vi "Modify_Dot_Characterstic(Status)-2.vi"(0 "Dot matrix IN":i16[][](array[numeric]), 1 "X2":dbl, 2 "Y2":dbl, 5 "Frame-to-frame displ":dbl[][](array[numeric]), 7 "Dot charact":i16, 9 "multipler":i32=4, 11 "error IN":errorcluster, 12 "# column":i32, 13 "Size Rows":i32) -> (4 "Dot matrix OUT":i16[][](array[numeric]), 15 "error OUT":errorcluster)   [LabVIEW 2013]
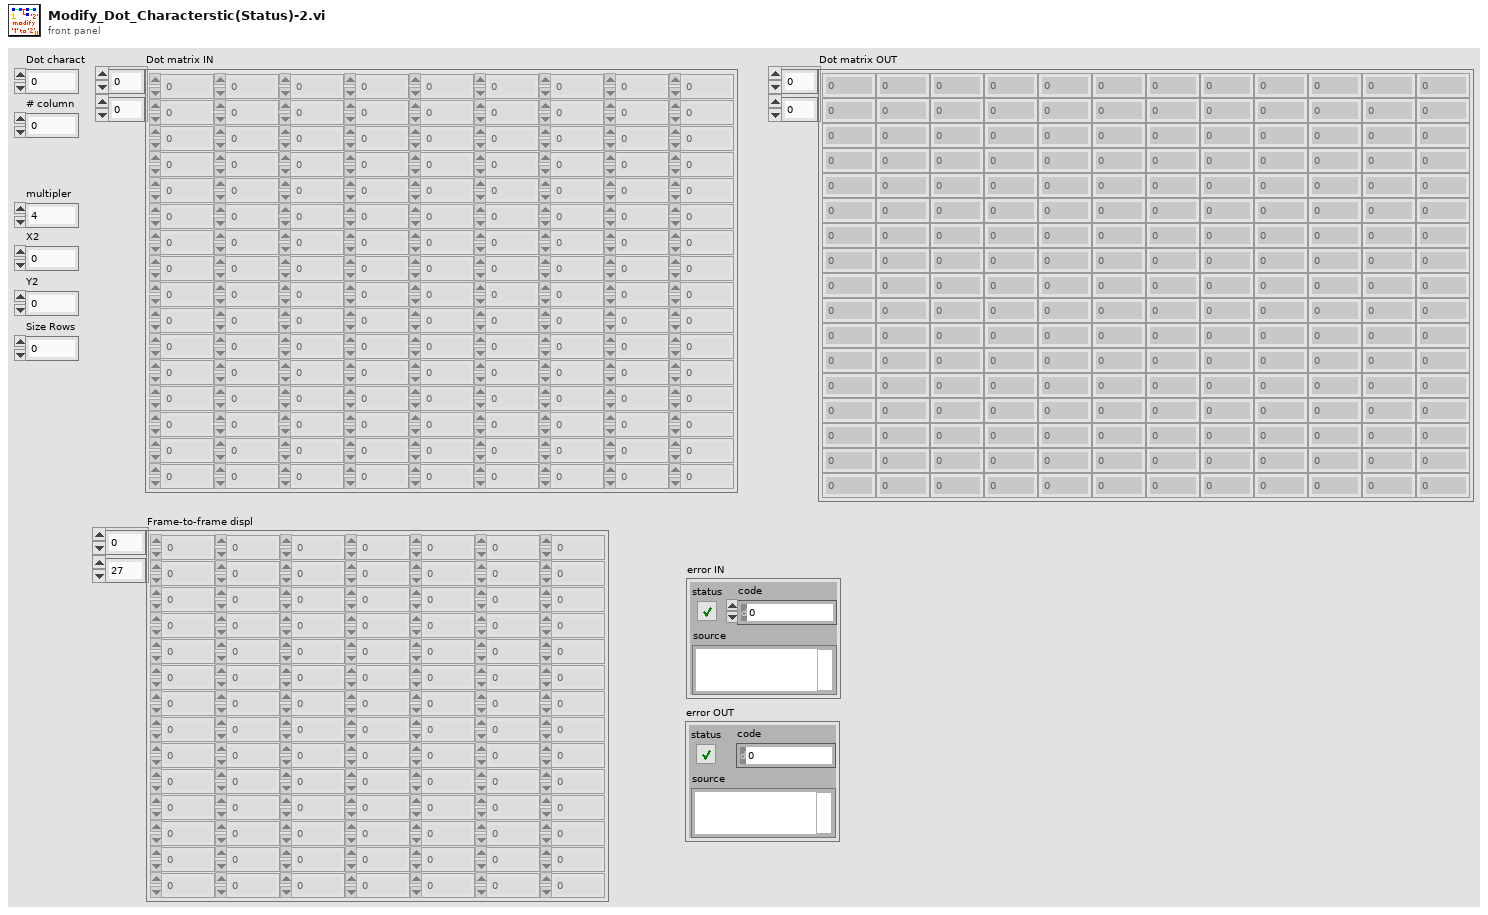
[diagram p1: front panel]
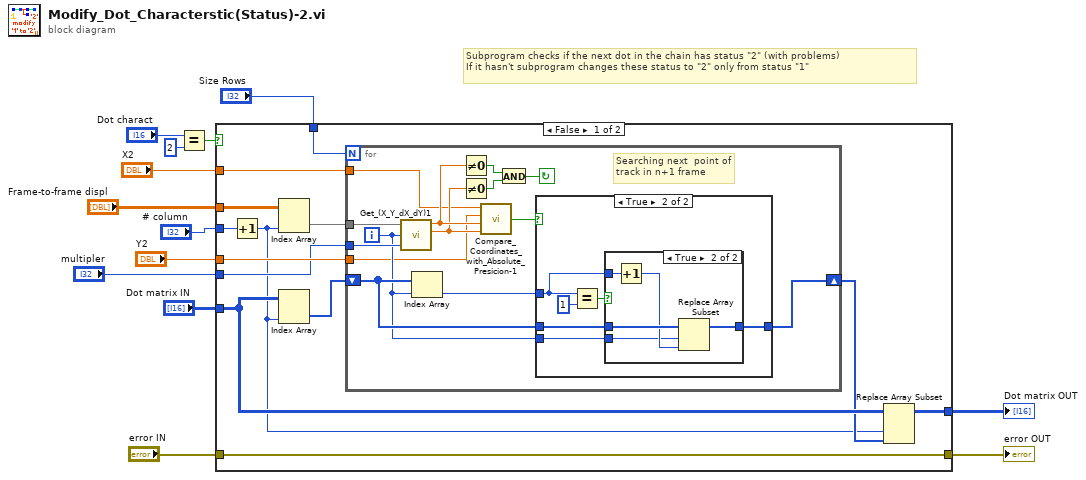
[diagram p0: block diagram]
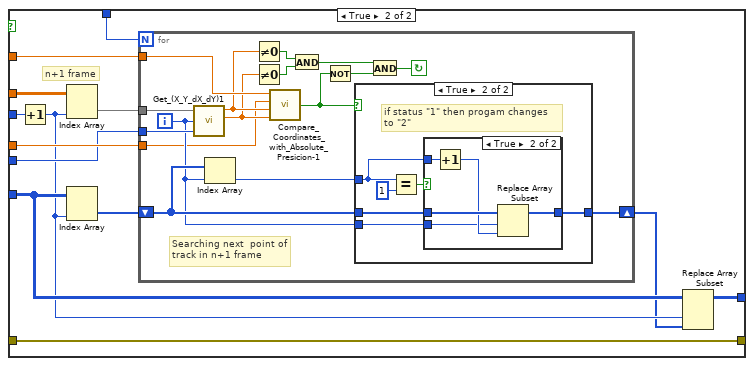
[diagram p4: hidden frame]
diagram:
  # "Subprogram checks if the next dot in the chain has status \"2\" (with problems)\nIf it hasn't subprogram changes these status to \"2\" only from status \"1\""
  n1 = Equal?(x="Dot charact", y=i16 2) -> (x = y?=w11:bool)
  n2 = case shown="False" w11 {
    tunnel: "Dot matrix IN" -> [w18 w58]
    tunnel: "# column" -> [w24 w66]
    tunnel: "multipler" -> [w20 w61]
    tunnel: "X2" -> [w23 w65]
    tunnel: "Frame-to-frame displ" -> [w25 w64]
    tunnel: "Y2" -> [w21 w62]
    tunnel: "Size Rows" -> [w26 w59]
    tunnel: [w15 w55] -> w2
    tunnel: "error IN" -> [w14 w54]
    tunnel: [w14 w54] -> w1
    frame False {
      n3 = Increment(x=w24) -> (x+1=w16:i32)
      n4 = Index Array(array=w25, index (col)=w16) -> (element=w22:dbl[])  [unwired: 1 in]
      n5 = Index Array(array=w18, index (col)=w16) -> (element=w19:i16[])  [unwired: 1 in]
      n6 = for {
        N: w26 -> [_]
        tunnel: w20 -> [w37]
        tunnel: w22 -> [w40]
        tunnel: w23 -> [w29]
        tunnel: w21 -> [w28]
        shift-right: [w33] -> w17
        shift-left: w19 -> [w35]
        i -> [w34]
        stop <- w32 continue-if-true
        # "Searching next  point of track in n+1 frame"
        n7 = call "Get_(X_Y_dX_dY)1.vi"("(X,Y,dX,dY)"=w40, "index"=w34, "multiplier"=w37) -> ("X"=w31:dbl, "Y"=w30:dbl)  [unwired: 2 out]
        n8 = Index Array(array=w35, index=w34) -> (element=w36:i16)
        n9 = Not Equal To 0?(x=w31) -> (x != 0?=w39:bool)
        n10 = Not Equal To 0?(x=w30) -> (x != 0?=w38:bool)
        n11 = call "Compare_Coordinates_with_Absolute_Presicion-1.vi"("X 1"=w29, "Y 1"=w28, "X 2"=w31, "Y 2"=w30) -> ("[OUT] Same coordinates?"=w27:bool)  [unwired: 1 in]
        n12 = And(x=w39, y=w38) -> (x .and. y?=w32:bool)
        n13 = case shown="True" w27 {
          tunnel: w36 -> [_ w45]
          tunnel: w35 -> [w41 w44]
          tunnel: w34 -> [_ w43]
          tunnel: [w41 w42] -> w33
          frame False {
          }
          frame True {
            n14 = Equal?(x=w45, y=i16 1) -> (x = y?=w46:bool)
            n15 = case shown="True" w46 {
              tunnel: w45 -> [_ w53]
              tunnel: w44 -> [w48 w52]
              tunnel: w43 -> [_ w50]
              tunnel: [w48 w49] -> w42
              frame False {
              }
              frame True {
                n16 = Increment(x=w53) -> (x+1=w51:i16)
                n17 = Replace Array Subset(array=w52, new element=w51, index=w50) -> (w49:i16[])
              }
            }
          }
        }
      }
      n18 = Replace Array Subset(array=w18, new element=w17, index (col)=w16) -> (w15:i16[][])  [unwired: 1 in]
    }
    frame True {
      # "n+1 frame"
      n19 = Increment(x=w66) -> (x+1=w57:i32)
      n20 = Index Array(array=w64, index (col)=w57) -> (element=w63:dbl[])  [unwired: 1 in]
      n21 = Index Array(array=w58, index (col)=w57) -> (element=w60:i16[])  [unwired: 1 in]
      n22 = for {
        N: w59 -> [_]
        tunnel: w61 -> [w79]
        tunnel: w63 -> [w82]
        tunnel: w65 -> [w71]
        tunnel: w62 -> [w68]
        shift-right: [w72] -> w56
        shift-left: w60 -> [w75]
        i -> [w74]
        stop <- w77 continue-if-true
        # "Searching next  point of track in n+1 frame"
        n23 = call "Get_(X_Y_dX_dY)1.vi"("(X,Y,dX,dY)"=w82, "index"=w74, "multiplier"=w79) -> ("X"=w70:dbl, "Y"=w69:dbl)  [unwired: 2 out]
        n24 = Index Array(array=w75, index=w74) -> (element=w76:i16)
        n25 = Not Equal To 0?(x=w70) -> (x != 0?=w81:bool)
        n26 = Not Equal To 0?(x=w69) -> (x != 0?=w80:bool)
        n27 = call "Compare_Coordinates_with_Absolute_Presicion-1.vi"("X 1"=w71, "Y 1"=w68, "X 2"=w70, "Y 2"=w69) -> ("[OUT] Same coordinates?"=w67:bool)  [unwired: 1 in]
        n28 = And(x=w81, y=w80) -> (x .and. y?=w78:bool)
        n29 = Not(x=w67) -> (.not. x?=w73:bool)
        n30 = case shown="True" w67 {
          tunnel: w76 -> [_ w87]
          tunnel: w75 -> [w83 w86]
          tunnel: w74 -> [_ w85]
          tunnel: [w83 w84] -> w72
          frame False {
          }
          frame True {
            # "if status \"1\" then progam changes \nto \"2\""
            n31 = Equal?(x=w87, y=i16 1) -> (x = y?=w88:bool)
            n32 = case shown="True" w88 {
              tunnel: w87 -> [_ w95]
              tunnel: w86 -> [w90 w94]
              tunnel: w85 -> [_ w92]
              tunnel: [w90 w91] -> w84
              frame False {
              }
              frame True {
                n33 = Increment(x=w95) -> (x+1=w93:i16)
                n34 = Replace Array Subset(array=w94, new element=w93, index=w92) -> (w91:i16[])
              }
            }
          }
        }
        n35 = And(x=w78, y=w73) -> (x .and. y?=w77:bool)
      }
      n36 = Replace Array Subset(array=w58, new element=w56, index (col)=w57) -> (w55:i16[][])  [unwired: 1 in]
    }
  }
  "Dot matrix OUT" <- w2
  "error OUT" <- w1
